vi "run_experiment_sCMOS_DAC_pre_refactor.vi"() -> ()   [LabVIEW 2015]
uses:
  <vilib>/DAQmx/write.llb/DAQmx Write (Digital Bool 1Line 1Point).vi
  <vilib>/DAQmx/read.llb/DAQmx Read (Analog 1D Wfm NChan NSamp).vi
  <vilib>/DAQmx/read.llb/DAQmx Read (Digital 2D U32 NChan NSamp).vi
  <vilib>/DAQmx/write.llb/DAQmx Write (Digital 1D Wfm NChan NSamp).vi
  <vilib>/DAQmx/write.llb/DAQmx Write (Analog Wfm 1Chan NSamp).vi
  <vilib>/DAQmx/create/channels.llb/DAQmx Create Channel (DO-Digital Output).vi
  <vilib>/DAQmx/miscellaneous.llb/DAQmx Fill In Error Info.vi
  <vilib>/Utility/file.llb/Write Delimited Spreadsheet (DBL).vi
  <vilib>/Waveform/DWDTOps.llb/DWDT Uncompress Digital.vi
  <vilib>/addons/h5labview2/file/H5F.lvlib
panel:
  out "SampClk.Rate":dbl
  out "Num Stimuli":i32
  out "V Offset":i32
  out "H Offset":i32
  out "Digital Error":errorcluster
  out "Analog Error":errorcluster
  out "ms between stimuli":i32=2500
  out "Rep":i32
  out "DO Samps Written":u32
  out ".dcimg --> .tiff":bool
  out ".dcimg count":i32
  in  "Use .dcimg":bool
  out "# tiffs":i32
  in  "Use Tiffs":bool
  in  "Configure Cam":bool
  out "Stimulus Order":i32[](array[numeric])
  in  "Randomize":bool
  out "Stop Input":bool
  out "AO Samps Written":u32
  out "temp .dcimg filepath":path
  out "Exposure":dbl
  out "V Width":i32
  out "H Width":i32
  out "Acquiring Frames":bool
  out "Cumulative Frames":i32
  out "Display":T1(plugin-control)
  out "DAC Input":waveform(dbl)[](graph) caption="DAC Input Display"
  out "error out":errorcluster
  out "Current Stimulus Name":string
  out "Current Piezo Command":waveform(dbl)(graph)
  out "Current Stim Frames":i32
  out "Current Stim Duration":dbl
  out "Current Stimulus Save Path":path
  in  "Number Reps":dbl
  out "Experiment Path":path
  out "Timestamp":string
  out "Genotype":string
  out "Fly Name":string
  out "Experiment Name":string
  in  "Metadata Path":path
  out "Stimulus Files":path[](array[path])
  out "Protocol Name":string
  out "Protocol Rate (Hz)":i32
  in  "Protocol Path":path
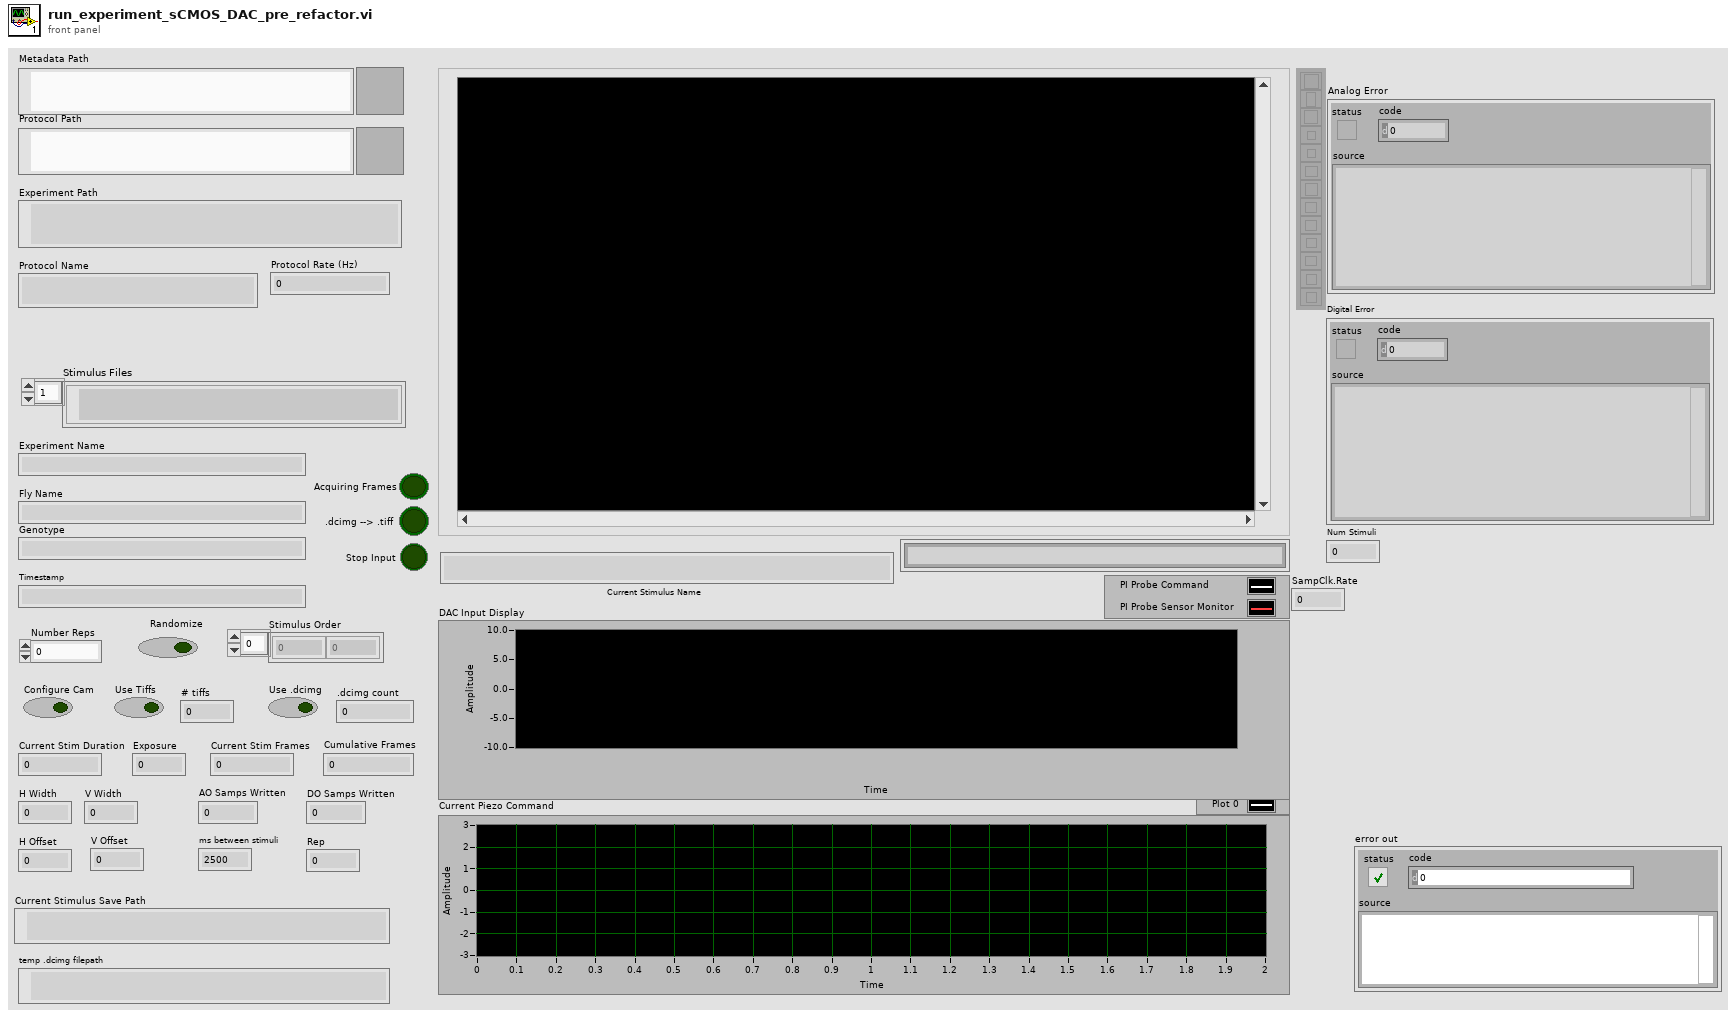
[diagram p1: front panel]
types:
  T1 = typedef "IMAQ Image.ctl" = refnum<image>
  T2 = cluster{"Value":i32, "Minimum":i32, "Maximum":i32, "Increment":i32}
  T3 = cluster{"Rows Per Strip":i32, "Photometric":i32, "Compression Type":i32}
  T4 = typedef "Image Type" = u32
  T5 = cluster{"height":u32, "width":u32, "datatype":u32}
  T6 = cluster{"piezo_command":dbl[], "alignment_command":dbl[]}
  T7 = cluster{"piezo_cmd":i32, "piezo_sensor":i32, "cam_trig_1":i32, "cam_trig_2":i32, "alignment_cmd":i32}
  T8 = typedef "hid_t.ctl" = i32
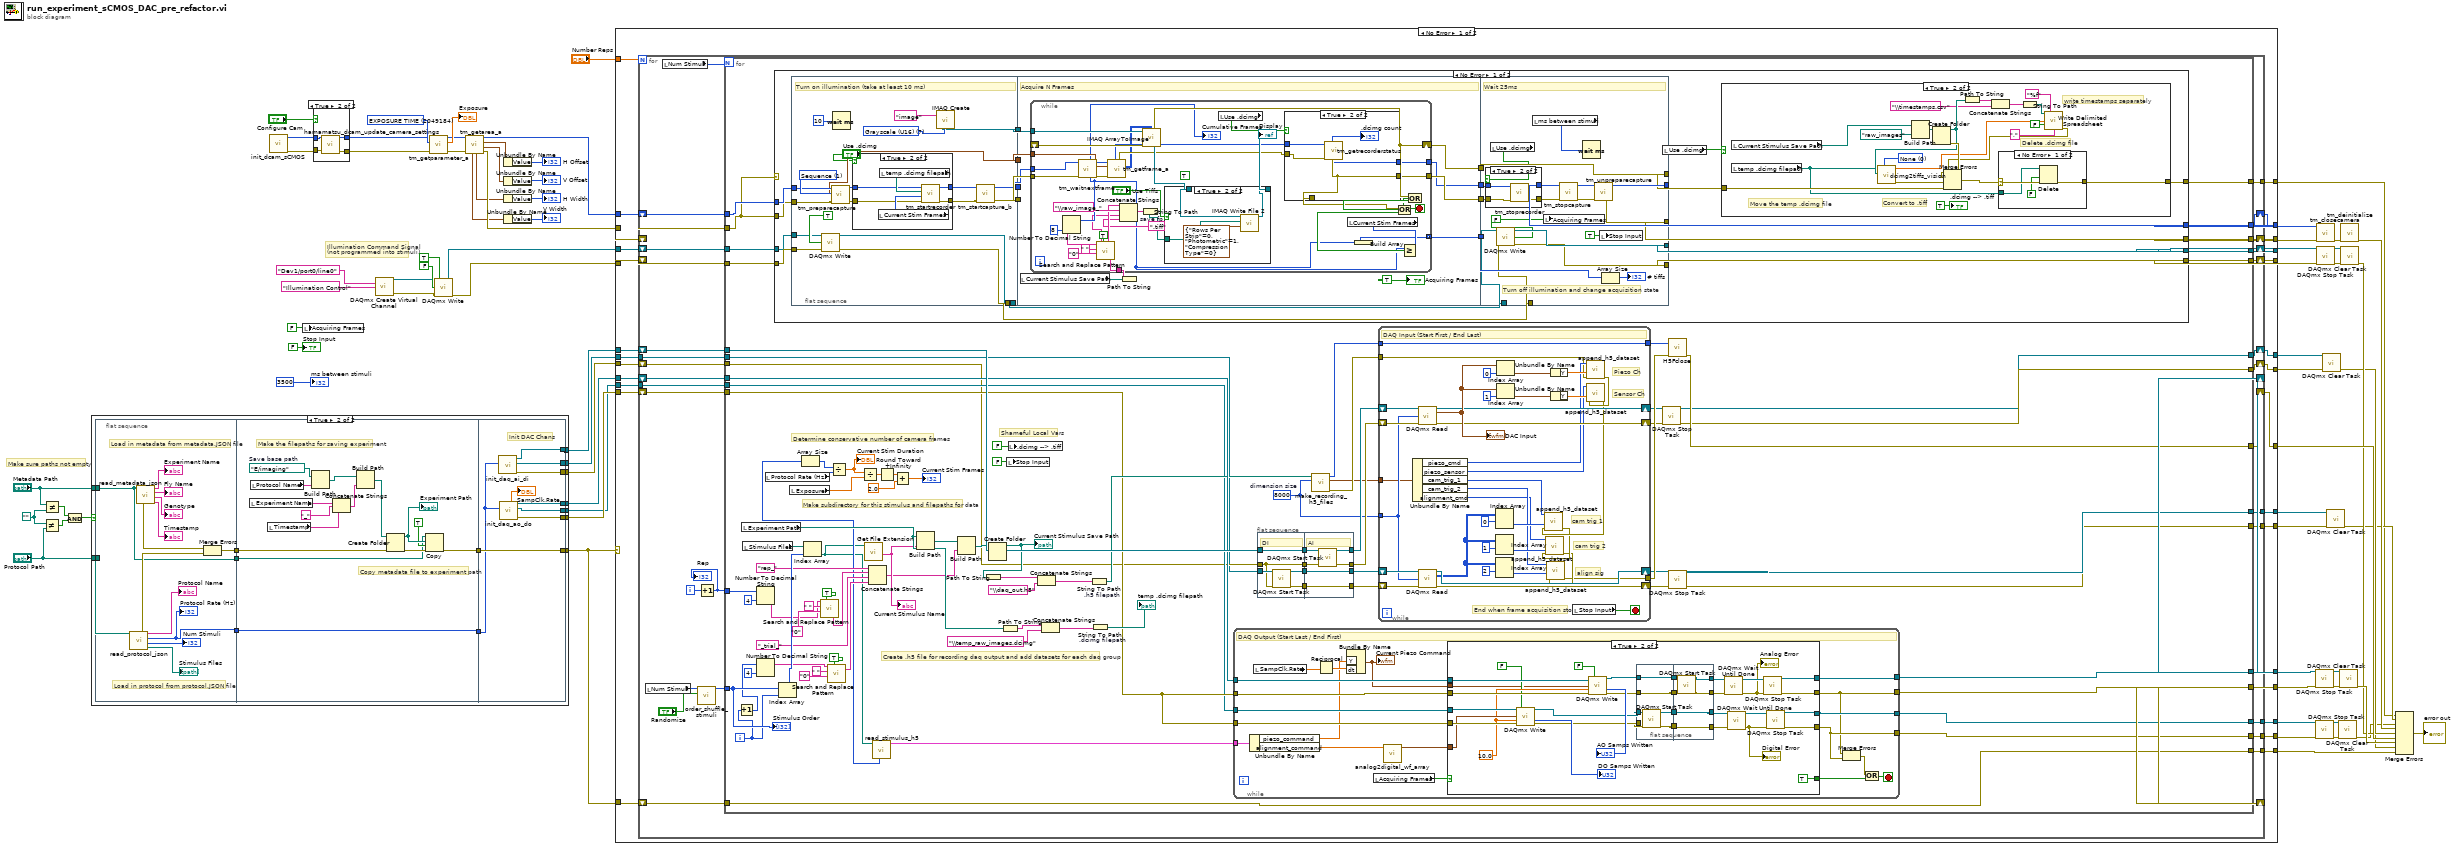
[diagram p0: block diagram]
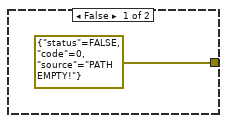
[diagram p3: hidden frame]
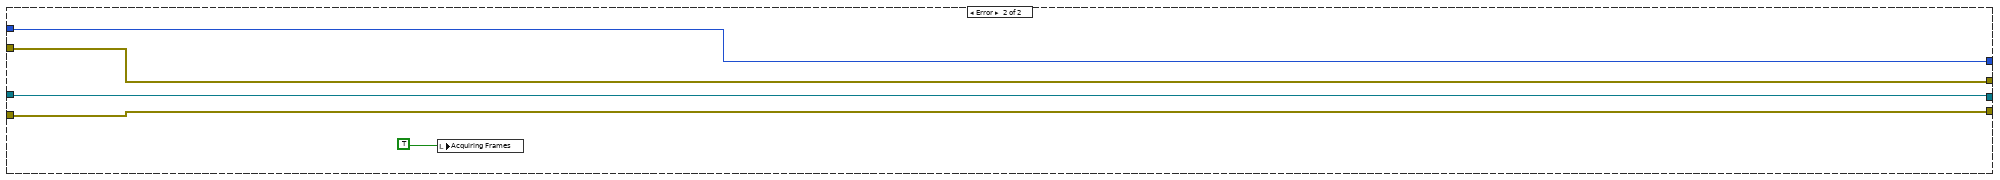
[diagram p10: hidden frame]
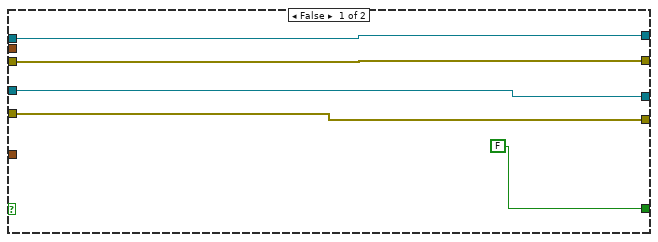
[diagram p11: hidden frame]
diagram:
  w24 = u32 2049184 items=["SENSOR MODE"=4212128, "CCD MODE"=4212384, "READOUT MODE"=4211872, "ACTIVE VIEW INDEX"=4343136, "BITS PER CHANNEL"=4342976, "IMAGE PIXEL TYPE"=4343296, "BINNING"=4215968, "EXPOSURE TIME"=2049184, "CONTRAST GAIN"=3163312, "CONTRAST OFFSET"=3163328, "LIGHT MODE"=2114720, "SENSITIVITY"=2114992, "PHOTON IMAGING MODE"=2115200, "HIGH DYNAMIC RANGE MODE"=3163360, "WHITE BALANCE"=3163568, "TEMPERATURE"=2115232, "TEMPERATURE TARGET"=2115264, "SENSOR COOLER FAN"=2115296, "LINEBUNDLE HEIGHT"=4212192, "MECHANICAL SHUTTER"=2115488, "BACK FOCUS POSITION"=8422304, "TRIGGER CONNECTOR"=1066432, "TRIGGER SOURCE"=1066144, "OUTPUT TRIGGER SOURCE"=1852576, "TRIGGER GLOBAL EXPOSURE"=2049680, "FIRST TRIGGER BEHAVIOR"=2049696, "CHANNEL SYNC"=1852352, "READOUT DIRECTION"=4211904, "PRE HSYNC COUNT"=1852704] ("Parameter")
  w4 = path ""
  # "Make sure paths not empty"
  # "Illumination Command Signal \n(not programmed into stimuli)"
  n1 = Not Equal?(x=w4, y="Protocol Path") -> (x != y?=w6:bool)
  n2 = Not Equal?(x="Metadata Path", y=w4) -> (x != y?=w7:bool)
  n3 = And(x=w7, y=w6) -> (x .and. y?=w34:bool)
  n4 = case shown="True" w34 {
    tunnel: [errorcluster {"status"=FALSE, "code"=0, "source"="PATH EMPTY!"} ("error out") w86] -> w42
    tunnel: "Metadata Path" -> [_ w85]
    tunnel: "Protocol Path" -> [_ w84]
    tunnel: [_ w80] -> w38
    tunnel: [_ w79] -> w37
    tunnel: [_ w78] -> w36
    tunnel: [_ w77] -> w35
    tunnel: [_ w76] -> w33
    tunnel: [_ w75] -> w27
    frame False {
    }
    frame True {
      n5 = flat-sequence {
        tunnel: [w93] -> w88
        tunnel: [w92] -> w87
        tunnel: w85 -> [w92]
        tunnel: w84 -> [w91]
        tunnel: [w90] -> w81
        tunnel: w88 -> [w105]
        tunnel: w87 -> [w104]
        tunnel: [w103] -> w83
        tunnel: [w102] -> w82
        tunnel: w81 -> [w102]
        tunnel: [w125] -> w86
        tunnel: w83 -> [w125]
        tunnel: w82 -> [w122]
        tunnel: [w124] -> w80
        tunnel: [w123] -> w79
        tunnel: [w121] -> w78
        tunnel: [w119] -> w77
        tunnel: [w120] -> w76
        tunnel: [w118] -> w75
        frame #0 {
          # "Load in metadata from metadata.JSON file"
          # "Load in protocol from protocol.JSON file"
          n6 = call "read_protocol_json.vi"("Path"=w91) -> ("stims"=→"Stimulus Files":path[], "n_stims"=→"Num Stimuli":i32, "rate"=w90:i32, "protocol name"=→"Protocol Name":string, "error out"=w95:errorcluster)  [unwired: 6 in]
          "Protocol Rate (Hz)" <- w90
          n7 = call "read_metadata_json.vi"("Path"=w92) -> ("exp_time"=→"Timestamp":string, "genotype"=→"Genotype":string, "fly_name"=→"Fly Name":string, "exp_ name"=→"Experiment Name":string, "error out"=w94:errorcluster)  [unwired: 6 in]
          n8 = Merge Errors(w94, w95) -> (w93:errorcluster)
        }
        frame #1 {
          w112 = path "E:/imaging"  # Save base path
          # "Copy metadata file to experiment path"
          # "Make the filepaths for saving experiment"
          n9 = local read "Experiment Name"() -> (w109:string)
          n10 = local read "Protocol Name"() -> (w111:string)
          n11 = local read "Timestamp"() -> (w107:string)
          n12 = Build Path(base path=w112, name or relative path=w111) -> (appended path=w110:path)
          n13 = Concatenate Strings(w109, "_", w107) -> (w106:string)
          n14 = Build Path(base path=w110, name or relative path=w106) -> (appended path=w113:path)
          n15 = Create Folder(path (use dialog)=w113, error in=w105) -> (created path=w116:path, error out=w115:errorcluster)  [unwired: 1 in, 1 out]
          "Experiment Path" <- w116
          n16 = Copy(8:w115, 9:TRUE ("overwrite (F)"), 10:w116, 11:w104) -> (0:w103:errorcluster)  [unwired: 1 in, 2 out]
        }
        frame #2 {
          # "Init DAC Chans"
          n17 = call "init_daq_ai_di.vi"("Sample Rate"=w122) -> ("error out"=w123:errorcluster, "DI Out"=w118:refnum<k21>, "AI Out"=w124:refnum<k21>)  [unwired: 7 in, 1 out]
          n18 = call "init_daq_ao_do.vi"("Rate"=w122) -> ("error out"=w119:errorcluster, "DO Out"=w120:refnum<k21>, "AO Out"=w121:refnum<k21>, "SampClk.Rate"=→"SampClk.Rate":dbl)  [unwired: 7 in]
        }
      }
    }
  }
  n19 = call "init_dcam_sCMOS.vi"() -> ("error out"=w2:errorcluster, "Handle out"=w3:u32)  [unwired: 10 in]
  n20 = local write "Acquiring Frames"(FALSE ("Acquiring Frames")) -> ()
  n21 = case shown="True" "Configure Cam" {
    tunnel: [w126 w131] -> w15
    tunnel: [w127 w130] -> w14
    tunnel: w3 -> [w127 w129]
    tunnel: w2 -> [w126 w128]
    frame False {
    }
    frame True {
      n22 = call "hamamatsu_dcam_update_camera_settings.vi"("error in (no error)"=w128, "Handle in"=w129) -> ("error out"=w131:errorcluster, "Handle out"=w130:u32)  [unwired: 6 in]
    }
  }
  n23 = call-poly <vilib>:"DAQmx Create Virtual Channel.vi"("lines"=tag "Dev1/port0/line0" ("DAQmx Physical Channel"), "name to assign"="Illumination Control") -> ("task out"=w44:refnum<k21>, "error out"=w43:errorcluster)  [unwired: 12 in]
  n24 = call <userlib>:"tm_getparameter_a.vi"("error in (no error)"=w15, "Parameter"=w24, "Handle in"=w14) -> ("error out"=w19:errorcluster, "Value out"=→"Exposure":dbl, "Handle out"=w18:u32)  [unwired: 6 in]
  n25 = call-poly <vilib>:"DAQmx Write.vi"("task/channels in"=w44, "auto start"=TRUE, "data"=FALSE, "error in"=w43) -> ("task out"=w50:refnum<k21>, "error out"=w49:errorcluster)  [unwired: 9 in, 1 out]
  n26 = call <userlib>:"tm_getarea_a.vi"("error in (no error)"=w19, "Handle in"=w18) -> ("error out"=w46:errorcluster, "V Offset"=w22:T2, "H Offset"=w23:T2, "Handle out"=w47:u32, "H Width"=w21:T2, "V Width"=w20:T2)  [unwired: 4 in]
  n27 = Unbundle By Name(w23) -> ("Value"=→"H Offset":i32)
  n28 = Unbundle By Name(w22) -> ("Value"=→"V Offset":i32)
  n29 = Unbundle By Name(w21) -> ("Value"=→"H Width":i32)
  n30 = Unbundle By Name(w20) -> ("Value"=→"V Width":i32)
  n31 = case shown="No Error" w42 {
    tunnel: w47 -> [w158 w562]
    tunnel: w46 -> [w157 w561]
    tunnel: [w151 _] -> w58
    tunnel: [w150 _] -> w59
    tunnel: [w156 _] -> w62
    tunnel: [w155 _] -> w63
    tunnel: [w154 w561] -> w55
    tunnel: [w153 w562] -> w54
    tunnel: [w152 _] -> w61
    tunnel: [w149 _] -> w53
    tunnel: [w148 _] -> w52
    tunnel: w50 -> [w147 _]
    tunnel: w49 -> [w146 _]
    tunnel: w38 -> [w145 _]
    tunnel: w37 -> [w144 _]
    tunnel: w36 -> [w143 _]
    tunnel: w35 -> [w142 _]
    tunnel: [w141 _] -> w11
    tunnel: w42 -> [w140 _]
    tunnel: [w139 _] -> w41
    tunnel: w33 -> [w138 _]
    tunnel: [w137 _] -> w28
    tunnel: [w136 _] -> w29
    tunnel: w27 -> [w135 _]
    tunnel: [w134 _] -> w26
    tunnel: [w133 _] -> w25
    tunnel: "Number Reps" -> [w132 _]
    frame No Error {
      n32 = for {
        N: w132 -> [_]
        tunnel: [w173] -> w141
        tunnel: [w171] -> w139
        shift-right: [w185] -> w153
        shift-left: w158 -> [w190]
        shift-right: [w186] -> w154
        shift-left: w157 -> [w189]
        shift-right: [w183] -> w151
        shift-left: w147 -> [w179]
        shift-right: [w182] -> w150
        shift-left: w146 -> [w178]
        shift-right: [w180] -> w148
        shift-left: w145 -> [w177]
        shift-right: [w181] -> w149
        shift-left: w144 -> [w176]
        shift-right: [w187] -> w155
        shift-left: w143 -> [w175]
        shift-right: [w184] -> w152
        shift-left: w142 -> [w174]
        shift-right: [w188] -> w156
        shift-left: w140 -> [w172]
        tunnel: w138 -> [w170]
        tunnel: [w169] -> w137
        tunnel: [w168] -> w136
        tunnel: w135 -> [w167]
        tunnel: [w166] -> w134
        tunnel: [w165] -> w133
        i -> [w160]
        n33 = local read "Num Stimuli"() -> (w163:i32)
        n34 = local read "Num Stimuli"() -> (w161:i32)
        n35 = call "order_shuffle_stimuli.vi"("Randomize?"="Randomize", "N Stimuli"=w163) -> ("Riffled"=w162:i32[])  [unwired: 9 in]
        n36 = Increment(x=w160) -> (x+1=w159:i32)
        "Rep" <- w159
        n37 = for {
          N: w161 -> [_]
          tunnel: w190 -> [w262]
          tunnel: w189 -> [w198]
          tunnel: [w276] -> w188
          tunnel: [w275] -> w187
          tunnel: [w248] -> w186
          tunnel: [w249] -> w185
          tunnel: [w271] -> w184
          tunnel: [w268] -> w183
          tunnel: [w267] -> w182
          tunnel: [w266] -> w181
          tunnel: [w265] -> w180
          tunnel: w179 -> [w250]
          tunnel: w178 -> [w251]
          tunnel: w177 -> [w264]
          tunnel: w176 -> [w210]
          tunnel: w175 -> [w263]
          tunnel: w174 -> [w216]
          tunnel: [w242] -> w173
          tunnel: w172 -> [w241]
          tunnel: [w241] -> w171
          tunnel: w162 -> [w230]
          tunnel: w159 -> [w191]
          tunnel: w170 -> [w215]
          tunnel: [w214] -> w169
          tunnel: [w213] -> w168
          tunnel: w167 -> [w209]
          tunnel: [w202] -> w166
          tunnel: [w201] -> w165
          i -> [w196]
          w194 = 8000  # dimension size
          # "Shameful Local Vars"
          # "Create .h5 file for recording daq output and add datasets for each daq group"
          # "Determine conservative number of camera frames"
          # "Make subdirectory for this stimulus and filepaths for data"
          n38 = Increment(x=w196) -> (x+1=w195:i32)
          n39 = local read "Experiment Path"() -> (w253:path)
          n40 = local read "Stimulus Files"() -> (w280:path[])
          n41 = Number To Decimal String(number=w191, width (-)=i16 4) -> (decimal integer string=w219:string)
          n42 = Number To Decimal String(number=w195, width (-)=i16 4) -> (decimal integer string=w223:string)
          n43 = local read "Protocol Rate (Hz)"() -> (w244:i32)
          n44 = case shown="No Error" w198 {
            tunnel: [w295 w453] -> w268
            tunnel: [w294 w452] -> w267
            tunnel: w262 -> [w305 w455]
            tunnel: w198 -> [w304 w454]
            tunnel: w251 -> [w303 w452]
            tunnel: w250 -> [w302 w453]
            tunnel: [w301 w455] -> w249
            tunnel: [w300 w454] -> w248
            tunnel: [w298 _] -> w242
            frame No Error {
              n45 = flat-sequence {
                tunnel: [w341] -> w312
                tunnel: [w355] -> w311
                tunnel: [w340] -> w310
                tunnel: [w352] -> w309
                tunnel: w305 -> [w357]
                tunnel: w304 -> [w356]
                tunnel: w303 -> [w350]
                tunnel: w302 -> [w349]
                tunnel: [w348] -> w293
                tunnel: [w347] -> w292
                tunnel: w312 -> [w377]
                tunnel: w311 -> [w376]
                tunnel: w310 -> [w375]
                tunnel: [w368] -> w308
                tunnel: [w374] -> w307
                tunnel: w309 -> [w373]
                tunnel: [w372] -> w306
                tunnel: [w369] -> w297
                tunnel: w308 -> [w433]
                tunnel: w307 -> [w434]
                tunnel: [w440] -> w300
                tunnel: [w442] -> w301
                tunnel: w306 -> [w444]
                tunnel: [w444] -> w299
                tunnel: w297 -> [w438]
                tunnel: [w430] -> w295
                tunnel: [w429] -> w294
                tunnel: w293 -> [w428]
                tunnel: w292 -> [w427]
                frame #0 {
                  w354 = T4 7 items=["Grayscale (U8)", "Grayscale (I16)", "Grayscale (SGL)", "Complex (CSG)", "RGB (U32)", "HSL (U32)", "RGB (U64)", "Grayscale (U16)"] ("Image Type")
                  w358 = 1 items=["Snap", "Sequence"] ("Capture mode")
                  # "Turn on illumination (take at least 10 ms)"
                  n46 = call-poly <vilib>:"DAQmx Write.vi"("task/channels in"=w349, "data"=TRUE, "error in"=w350) -> ("task out"=w348:refnum<k21>, "error out"=w347:errorcluster)  [unwired: 10 in, 1 out]
                  n47 = call <userlib>:"tm_preparecapture.vi"("error in (no error)"=w356, "Capture mode"=w358, "Handle in"=w357) -> ("error out"=w345:errorcluster, "Buffer Info"=w355:T5, "Handle out"=w344:u32)  [unwired: 5 in, 1 out]
                  n48 = Wait (ms)(milliseconds to wait=u32 10) -> ()  [unwired: 1 out]
                  n49 = case shown="True" "Use .dcimg" {
                    tunnel: [w361 w365] -> w343
                    tunnel: [w360 w364] -> w342
                    tunnel: w345 -> [w360 w363]
                    tunnel: w344 -> [w361 w362]
                    frame False {
                    }
                    frame True {
                      n50 = local read "Current Stim Frames"() -> (w366:i32)
                      n51 = local read "temp .dcimg filepath"() -> (w367:path)
                      n52 = call <userlib>:"tm_startrecorder.vi"("error in (no error)"=w363, "frames"=w366, "File"=w367, "Handle in"=w362) -> ("error out"=w364:errorcluster, "Handle out"=w365:u32)  [unwired: 6 in]
                    }
                  }
                  n53 = call "IMAQ Create"("Image Name"="image", "Image Type"=w354) -> ("New Image"=w352:T1)  [unwired: 3 in, 1 out]
                  n54 = call <userlib>:"tm_startcapture_b.vi"("error in (no error)"=w342, "Handle in"=w343) -> ("error out"=w341:errorcluster, "Handle out"=w340:u32)  [unwired: 8 in]
                }
                frame #1 {
                  # "Acquire N Frames"
                  n55 = local read "Current Stimulus Save Path"() -> (w371:path)
                  n56 = Path To String(path=w371) -> (string=w370:string)
                  n57 = while {
                    tunnel: w377 -> [w411]
                    tunnel: w376 -> [w410]
                    tunnel: w375 -> [w409]
                    tunnel: [w386] -> w368
                    tunnel: [w388] -> w374
                    tunnel: w373 -> [w407]
                    shift-right: [w404] -> w372
                    shift-left: _ -> [w406]
                    tunnel: w370 -> [w399]
                    tunnel: [w392] -> w369 mode=concatenating
                    stop <- w402 stop-if-true
                    (unwired) TRUE ("Reset")
                    n58 = call <userlib>:"tm_waitnextframe.vi"("error in (no error)"=w411, "Handle in"=w409) -> ("error out"=w413:errorcluster, "Frame Count"=w393:i32, "Handle out"=w412:u32)  [unwired: 6 in, 1 out]
                    "Cumulative Frames" <- w393
                    n59 = Number To Decimal String(number=w393, width (-)=i16 8) -> (decimal integer string=w381:string)
                    n60 = call <vilib>:"Search and Replace Pattern.vi"("string"=w381, "regular expression (\"\")"=" " ("regular expression (\"\")"), "replace string (\"\")"="0" ("replace string (\"\")"), "replace all? (F)"=TRUE) -> ("result string"=w380:string)  [unwired: 1 in, 1 out]
                    n61 = call <userlib>:"tm_getframe_a.vi"("error in (no error)"=w413, "Buffer Info"=w410, "Handle in"=w412) -> ("error out"=w389:errorcluster, "Data 16"=w379:u16[][], "Handle out"=w387:u32)  [unwired: 4 in, 2 out]
                    n62 = Concatenate Strings(w399, "\\raw_image_" ("string"), w380, ".tiff" ("string")) -> (w400:string)
                    n63 = String To Path "save fp"(string=w400) -> (path=w397:path)
                    n64 = call "IMAQ ArrayToImage"("Image Pixels (U16)"=w379, "error in (no error)"=w406, "Image"=w407) -> ("error out"=w404:errorcluster, "Image Out"=w398:T1)  [unwired: 7 in]
                    n65 = case shown="True" "Use Tiffs" {
                      tunnel: w398 -> [w421 w425]
                      tunnel: w397 -> [_ w424]
                      tunnel: [w421 w422] -> w396
                      frame False {
                      }
                      frame True {
                        n66 = call-poly "IMAQ Write File 2"("TIFF Options"=T3 {"Rows Per Strip"=0, "Photometric"=1, "Compression Type"=0}, "File Path"=w424, "Image"=w425) -> ("Image Out (duplicate)"=w422:T1)  [unwired: 7 in, 1 out]
                      }
                    }
                    "Display" <- w396
                    n67 = local read "Use .dcimg"() -> (w391:bool)
                    n68 = case shown="True" w391 {
                      tunnel: [w415 w419] -> w390
                      tunnel: w389 -> [w415 w420]
                      tunnel: [w415 w419] -> w388
                      tunnel: w387 -> [w414 w418]
                      tunnel: [w414 w417] -> w386
                      frame False {
                      }
                      frame True {
                        n69 = call <userlib>:"tm_getrecorderstatus.vi"("error in (no error)"=w420, "Handle"=w418) -> ("error out"=w419:errorcluster, "Count"=→".dcimg count":i32, "Handle"=w417:u32)  [unwired: 6 in, 1 out]
                      }
                    }
                    n70 = local read "Current Stim Frames"() -> (w408:i32)
                    n71 = Build Array(w393) -> (w392:i32[])
                    n72 = Greater Or Equal?(x=w393, y=w408) -> (x >= y?=w405:bool)
                    n73 = Or(x=w390, y=w405) -> (x .or. y?=w403:bool)
                    n74 = Or(x=w404, y=w403) -> (x .or. y?=w402:bool)
                  }
                  "Acquiring Frames" <- TRUE
                }
                frame #2 {
                  w426 = FALSE
                  # "Turn off illumination and change acquisition state"
                  # "Wait 25ms"
                  n75 = local read "Use .dcimg"() -> (w436:bool)
                  n76 = case shown="True" w436 {
                    tunnel: [w446 w449] -> w435
                    tunnel: w434 -> [w446 w450]
                    tunnel: w433 -> [w445 w447]
                    tunnel: [w445 w448] -> w432
                    frame False {
                    }
                    frame True {
                      n77 = call <userlib>:"tm_stoprecorder.vi"("error in (no error)"=w450, "Handle in"=w447) -> ("error out"=w449:errorcluster, "Handle out"=w448:u32)  [unwired: 8 in]
                    }
                  }
                  n78 = call-poly <vilib>:"DAQmx Write.vi"("task/channels in"=w428, "data"=w426, "error in"=w427) -> ("task out"=w430:refnum<k21>, "error out"=w429:errorcluster)  [unwired: 10 in, 1 out]
                  n79 = local read "ms between stimuli"() -> (w431:i32)
                  n80 = local write "Acquiring Frames"(w426) -> ()
                  n81 = call <userlib>:"tm_stopcapture.vi"("error in (no error)"=w435, "Handle in"=w432) -> ("error out"=w441:errorcluster, "Handle out"=w443:u32)  [unwired: 8 in]
                  n82 = Wait (ms)(milliseconds to wait=w431) -> ()  [unwired: 1 out]
                  n83 = call <userlib>:"tm_unpreparecapture.vi"("error in (no error)"=w441, "Handle in"=w443) -> ("error out"=w440:errorcluster, "Handle out"=w442:u32)  [unwired: 8 in]
                  n84 = local write "Stop Input"(TRUE ("Stop Input")) -> ()
                  n85 = Array Size(array=w438) -> (size(s)=→"# tiffs":i32)
                }
              }
              n86 = local read "Use .dcimg"() -> (w296:bool)
              n87 = case shown="True" w296 {
                tunnel: w299 -> [w313 w325]
                tunnel: [w313 w326] -> w298
                frame False {
                }
                frame True {
                  w330 = 0 items=["None", "JPEG", "Run Length Encoded", "Zip"] ("Compression Type")
                  # "write timestamps separately"
                  # "Delete .dcimg file"
                  # "Convert to .tiff"
                  # "Move the temp .dcimg file"
                  n88 = local read "Current Stimulus Save Path"() -> (w333:path)
                  n89 = local read "temp .dcimg filepath"() -> (w314:path)
                  n90 = Build Path(base path=w333, name or relative path=path "raw_images") -> (appended path=w331:path)
                  n91 = Create Folder(path (use dialog)=w331) -> (created path=w324:path, error out=w329:errorcluster)  [unwired: 2 in, 1 out]
                  n92 = call "dcimg2tiffs_vision.vi"("Compression Type"=w330, ".tiff Path"=w324, "DCIMG Path"=w314) -> ("Error Out"=w334:errorcluster, "Timestamps"=w319:dbl[])  [unwired: 7 in]
                  n93 = Path To String(path=w324) -> (string=w323:string)
                  n94 = Concatenate Strings(w323, "\\timestamps.csv" ("string")) -> (w321:string)
                  n95 = String To Path(string=w321) -> (path=w320:path)
                  n96 = call-poly <vilib>:"Write Delimited Spreadsheet.vi"("file path (dialog if empty)"=w320, "format (%.3f)"="%f", "1D data"=w319, "append to file? (F)"=FALSE, "delimiter (\\t)"="," ("delimiter (\\t)")) -> ("error out"=w318:errorcluster)  [unwired: 9 in, 1 out]
                  n97 = Merge Errors(w318, w329, w334, w325) -> (w327:errorcluster)
                  n98 = case shown="No Error" w327 {
                    selector: w327 -> [w338 w339]
                    tunnel: [w337 w339] -> w326
                    tunnel: w314 -> [w335 _]
                    frame No Error {
                      n99 = Delete(path (use dialog)=w335, confirm (F)=FALSE, error in=w338) -> (error out=w337:errorcluster)  [unwired: 2 in, 2 out]
                    }
                    frame Error {
                    }
                  }
                  ".dcimg --> .tiff" <- TRUE ("Converting .tiff")
                }
              }
            }
            frame Error {
              n100 = local write "Acquiring Frames"(TRUE ("Acquiring Frames")) -> ()
            }
          }
          n101 = Index Array(array=w230, index=w196) -> (element=w234:i32)
          n102 = local read "Exposure"() -> (w192:dbl)
          n103 = Index Array(array=w280, index=w234) -> (element=w197:path)
          n104 = call <vilib>:"Search and Replace Pattern.vi"("string"=w219, "regular expression (\"\")"=" " ("regular expression (\"\")"), "replace string (\"\")"="0" ("replace string (\"\")"), "replace all? (F)"=TRUE) -> ("result string"=w218:string)  [unwired: 1 in, 1 out]
          n105 = call <vilib>:"Search and Replace Pattern.vi"("string"=w223, "regular expression (\"\")"=" " ("regular expression (\"\")"), "replace string (\"\")"="0" ("replace string (\"\")"), "replace all? (F)"=TRUE) -> ("result string"=w224:string)  [unwired: 1 in, 1 out]
          n106 = call <vilib>:"Get File Extension.vi"("file"=w197) -> ("filename without extension"=w236:string)  [unwired: 6 in, 4 out]
          "Current Stimulus Name" <- w236
          n107 = Concatenate Strings("rep_", w218, "_trial_", w224) -> (w233:string)
          n108 = call "read_stimulus_h5.vi"("Path"=w197) -> ("output cluster"=w200:T6, "piezo_command"=w199:i32[])  [unwired: 7 in, 2 out]
          n109 = Array Size(array=w199) -> (size(s)=w245:i32)
          n110 = Divide(x=w245, y=w244) -> (x/y=w243:dbl)
          "Current Stim Duration" <- w243
          n111 = Divide(x=w243, y=w192) -> (x/y=w279:dbl)
          n112 = Round Toward +Infinity(x=w279) -> (ceil(x): smallest int >= x=w278:dbl)
          n113 = Add(x=w278, y=2.0) -> (x+y=→"Current Stim Frames":dbl)
          n114 = Build Path(base path=w253, name or relative path=w236) -> (appended path=w257:path)
          n115 = Build Path(base path=w257, name or relative path=w233) -> (appended path=w258:path)
          n116 = Create Folder(path (use dialog)=w258) -> (created path=w247:path)  [unwired: 2 in, 2 out]
          "Current Stimulus Save Path" <- w247
          n117 = Path To String(path=w247) -> (string=w255:string)
          n118 = Path To String(path=w253) -> (string=w259:string)
          n119 = local write "Stop Input"(FALSE ("Stop Input")) -> ()
          n120 = local write ".dcimg --> .tiff"(FALSE ("Converting .tiff")) -> ()
          n121 = Concatenate Strings(w255, "\\daq_out.h5" ("string")) -> (w254:string)
          n122 = Concatenate Strings(w259, "\\temp_raw_images.dcimg" ("string")) -> (w261:string)
          n123 = String To Path ".h5 filepath"(string=w254) -> (path=w240:path)
          n124 = String To Path ".dcimg filepath"(string=w261) -> (path=→"temp .dcimg filepath":path)
          n125 = while {
            tunnel: w263 -> [w472]
            tunnel: [w473] -> w275
            tunnel: [w465] -> w276
            tunnel: w216 -> [w471]
            tunnel: w216 -> [w469]
            tunnel: w215 -> [w468]
            tunnel: [w467] -> w214
            tunnel: [w466] -> w213
            tunnel: w200 -> [w464]
            stop <- w470 stop-if-true
            # "DAQ Output (Start Last / End First)"
            n126 = Unbundle By Name(w464) -> ("piezo_command"=w459:dbl[], "alignment_command"=w463:dbl[])
            n127 = local read "SampClk.Rate"() -> (w461:dbl)
            n128 = Reciprocal(x=w461) -> (1/x=w460:dbl)
            n129 = Bundle By Name("Y"=w459, "dt"=w460) -> (w458:waveform(dbl))  [unwired: 1 in]
            "Current Piezo Command" <- w458
            n130 = local read "Acquiring Frames"() -> (w474:bool)
            n131 = call "analog2digital_wf_array.vi"("analog waveform"=w463) -> ("digital array"=w462:digitalwaveform[])  [unwired: 7 in, 3 out]
            n132 = case shown="True" w474 {
              tunnel: w471 -> [w478 w508]
              tunnel: w472 -> [w479 w509]
              tunnel: [w479 w511] -> w473
              tunnel: [w478 w510] -> w465
              tunnel: [FALSE ("Stop Input") TRUE ("Stop Input")] -> w456
              tunnel: w469 -> [w476 w506]
              tunnel: [w476 w503] -> w466
              tunnel: [w475 w504] -> w467
              tunnel: w468 -> [w475 w505]
              tunnel: w462 -> [_ w502]
              tunnel: w458 -> [_ w480]
              frame False {
              }
              frame True {
                w493 = 10.0 ("timeout")
                n133 = call-poly <vilib>:"DAQmx Write.vi"("task/channels in"=w505, "auto start"=FALSE, "data"=w502, "timeout"=w493, "error in"=w506) -> ("task out"=w487:refnum<k21>, "number of samples written per channel"=→"DO Samps Written":u32, "error out"=w488:errorcluster)  [unwired: 8 in]
                n134 = call-poly <vilib>:"DAQmx Write.vi"("task/channels in"=w509, "auto start"=FALSE, "data"=w480, "timeout"=w493, "error in"=w508) -> ("task out"=w481:refnum<k21>, "number of samples written per channel"=→"AO Samps Written":u32, "error out"=w484:errorcluster)  [unwired: 8 in]
                n135 = flat-sequence {
                  tunnel: w488 -> [w517]
                  tunnel: w487 -> [w516]
                  tunnel: [w515] -> w501
                  tunnel: [w514] -> w500
                  tunnel: [w513] -> w499
                  tunnel: w484 -> [w513]
                  tunnel: w481 -> [w512]
                  tunnel: [w512] -> w498
                  tunnel: [w522] -> w485
                  tunnel: [w523] -> w486
                  tunnel: w501 -> [w523]
                  tunnel: w500 -> [w522]
                  tunnel: w499 -> [w521]
                  tunnel: [w520] -> w483
                  tunnel: [w519] -> w482
                  tunnel: w498 -> [w518]
                  frame #0 {
                    n136 = call <vilib>:"DAQmx Start Task.vi"("task/channels in"=w516, "error in"=w517) -> ("task out"=w515:refnum<k21>, "error out"=w514:errorcluster)  [unwired: 12 in]
                  }
                  frame #1 {
                    n137 = call <vilib>:"DAQmx Start Task.vi"("task/channels in"=w518, "error in"=w521) -> ("task out"=w519:refnum<k21>, "error out"=w520:errorcluster)  [unwired: 12 in]
                  }
                }
                n138 = call <vilib>:"DAQmx Wait Until Done.vi"("task/channels in"=w482, "error in"=w483) -> ("task out"=w496:refnum<k21>, "error out"=w495:errorcluster)  [unwired: 12 in]
                "Analog Error" <- w495
                n139 = call <vilib>:"DAQmx Wait Until Done.vi"("task/channels in"=w486, "error in"=w485) -> ("task out"=w491:refnum<k21>, "error out"=w490:errorcluster)  [unwired: 12 in]
                "Digital Error" <- w490
                n140 = call <vilib>:"DAQmx Stop Task.vi"("task/channels in"=w496, "error in"=w495) -> ("task out"=w511:refnum<k21>, "error out"=w510:errorcluster)  [unwired: 12 in]
                n141 = call <vilib>:"DAQmx Stop Task.vi"("task/channels in"=w491, "error in"=w490) -> ("task out"=w504:refnum<k21>, "error out"=w503:errorcluster)  [unwired: 12 in]
              }
            }
            n142 = Merge Errors(w465, w466) -> (w457:errorcluster)
            n143 = Or(x=w457, y=w456) -> (x .or. y?=w470:bool)
          }
          n144 = flat-sequence {
            tunnel: w264 -> [w282]
            tunnel: w210 -> [w281]
            tunnel: w209 -> [w283]
            tunnel: [w282] -> w208
            tunnel: [w281] -> w207
            tunnel: [w285] -> w206
            tunnel: [w284] -> w205
            tunnel: [w290] -> w211
            tunnel: [w291] -> w212
            tunnel: [w288] -> w273
            tunnel: [w289] -> w274
            tunnel: w208 -> [w286]
            tunnel: w207 -> [w287]
            tunnel: w206 -> [w291]
            tunnel: w205 -> [w290]
            frame #0 {
              # "DI"
              n145 = call <vilib>:"DAQmx Start Task.vi"("task/channels in"=w283, "error in"=w281) -> ("task out"=w284:refnum<k21>, "error out"=w285:errorcluster)  [unwired: 12 in]
            }
            frame #1 {
              # "AI"
              n146 = call <vilib>:"DAQmx Start Task.vi"("task/channels in"=w286, "error in"=w287) -> ("task out"=w289:refnum<k21>, "error out"=w288:errorcluster)  [unwired: 12 in]
            }
          }
          n147 = call "make_recording_h5_files.vi"("write/append size"=w194, "Path"=w240) -> ("error out"=w239:errorcluster, "dataset cluster"=w193:T7, "ref out"=w237:T8)  [unwired: 7 in]
          n148 = while {
            tunnel: w239 -> [w529]
            tunnel: [w524] -> w272
            shift-right: [w553] -> w270
            shift-left: w274 -> [w560]
            shift-right: [w552] -> w269
            shift-left: w273 -> [w559]
            tunnel: [w551] -> w238
            tunnel: w237 -> [w551]
            shift-right: [w546] -> w203
            shift-left: w212 -> [w548]
            shift-right: [w547] -> w204
            shift-left: w211 -> [w549]
            tunnel: w194 -> [w538]
            tunnel: w193 -> [w537]
            stop <- w550 stop-if-true
            # "cam trig 2"
            # "align sig"
            # "Sensor Ch"
            # "cam trig 1"
            # "Piezo Ch"
            # "End when frame acquisition stops"
            # "DAQ Input (Start First / End Last)"
            n149 = Unbundle By Name(w537) -> ("piezo_cmd"=w536:i32, "piezo_sensor"=w535:i32, "cam_trig_1"=w534:i32, "cam_trig_2"=w532:i32, "alignment_cmd"=w531:i32)
            n150 = call-poly <vilib>:"DAQmx Read.vi"("task/channels in"=w560, "number of samples per channel"=w538, "error in"=w559) -> ("task out"=w553:refnum<k21>, "data"=w554:waveform(dbl)[], "error out"=w552:errorcluster)  [unwired: 10 in]
            "DAC Input" <- w554
            n151 = call-poly <vilib>:"DAQmx Read.vi"("task/channels in"=w549, "number of samples per channel"=w538, "error in"=w548) -> ("task out"=w547:refnum<k21>, "data"=w542:u32[][], "error out"=w546:errorcluster)  [unwired: 10 in]
            n152 = Index Array(array=w542, index (row)=0 ("index")) -> (element=w533:u32[])  [unwired: 1 in]
            n153 = Index Array(array=w542, index (row)=1 ("index")) -> (element=w539:u32[])  [unwired: 1 in]
            n154 = Index Array(array=w542, index (row)=2 ("index")) -> (element=w530:u32[])  [unwired: 1 in]
            n155 = Index Array(array=w554, index=0) -> (element=w558:waveform(dbl))
            n156 = Index Array(array=w554, index=1) -> (element=w556:waveform(dbl))
            n157 = Unbundle By Name(w558) -> ("Y"=w541:dbl[])
            n158 = Unbundle By Name(w556) -> ("Y"=w540:dbl[])
            n159 = local read "Stop Input"() -> (w550:bool)
            n160 = call "append_h5_dataset.vi"("error in (no error)"=w529, "Data"=w541, "dset in"=w536) -> ("error out"=w528:errorcluster)  [unwired: 8 in]
            n161 = call "append_h5_dataset.vi"("error in (no error)"=w528, "Data"=w540, "dset in"=w535) -> ("error out"=w527:errorcluster)  [unwired: 8 in]
            n162 = call "append_h5_dataset.vi"("error in (no error)"=w527, "Data"=w533, "dset in"=w534) -> ("error out"=w526:errorcluster)  [unwired: 8 in]
            n163 = call "append_h5_dataset.vi"("error in (no error)"=w526, "Data"=w539, "dset in"=w531) -> ("error out"=w525:errorcluster)  [unwired: 8 in]
            n164 = call "append_h5_dataset.vi"("error in (no error)"=w525, "Data"=w530, "dset in"=w532) -> ("error out"=w524:errorcluster)  [unwired: 8 in]
          }
          n165 = call <vilib>:"DAQmx Stop Task.vi"("task/channels in"=w270, "error in"=w269) -> ("task out"=w265:refnum<k21>, "error out"=w266:errorcluster)  [unwired: 12 in]
          n166 = call <vilib>:"H5Fclose.vi"("error in (no error)"=w272, "ref"=w238) -> ("error out"=w271:errorcluster)  [unwired: 9 in]
          n167 = call <vilib>:"DAQmx Stop Task.vi"("task/channels in"=w204, "error in"=w203) -> ("task out"=w202:refnum<k21>, "error out"=w201:errorcluster)  [unwired: 12 in]
          "Stimulus Order" <- w230
        }
      }
    }
    frame Error {
    }
  }
  n168 = call <vilib>:"DAQmx Stop Task.vi"("task/channels in"=w63, "error in"=w62) -> ("task out"=w65:refnum<k21>, "error out"=w64:errorcluster)  [unwired: 12 in]
  n169 = call <vilib>:"DAQmx Stop Task.vi"("task/channels in"=w28, "error in"=w29) -> ("task out"=w32:refnum<k21>, "error out"=w31:errorcluster)  [unwired: 12 in]
  n170 = call <userlib>:"tm_closecamera.vi"("error in (no error)"=w55, "Handle in"=w54) -> ("error out"=w66:errorcluster)  [unwired: 9 in]
  n171 = call <vilib>:"DAQmx Stop Task.vi"("task/channels in"=w58, "error in"=w59) -> ("task out"=w68:refnum<k21>, "error out"=w67:errorcluster)  [unwired: 12 in]
  n172 = call <vilib>:"DAQmx Clear Task.vi"("task in"=w52, "error in"=w53) -> ("error out"=w51:errorcluster)  [unwired: 13 in]
  n173 = call <vilib>:"DAQmx Clear Task.vi"("task in"=w26, "error in"=w25) -> ("error out"=w12:errorcluster)  [unwired: 13 in]
  n174 = call <vilib>:"DAQmx Clear Task.vi"("task in"=w32, "error in"=w31) -> ("error out"=w30:errorcluster)  [unwired: 13 in]
  n175 = call <vilib>:"DAQmx Clear Task.vi"("task in"=w65, "error in"=w64) -> ("error out"=w60:errorcluster)  [unwired: 13 in]
  n176 = call <userlib>:"tm_deinitialize.vi"("error in (no error)"=w66) -> ("error out"=w56:errorcluster)  [unwired: 10 in]
  n177 = call <vilib>:"DAQmx Clear Task.vi"("task in"=w68, "error in"=w67) -> ("error out"=w57:errorcluster)  [unwired: 13 in]
  n178 = Merge Errors(w11, w12, w30, w56, w57, w61, w60, w51, w41) -> (→"error out":errorcluster)
  "Stop Input" <- FALSE ("Stop Input")
  "ms between stimuli" <- 3500 ("ms between stimuli")
